vi "Introduce Delay.vi"(8 "error in (no error)":errorcluster, 11 "Ms":u32=100) -> (0 "error out":errorcluster)   [LabVIEW 2018]
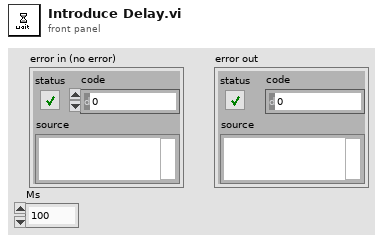
[diagram p1: front panel]
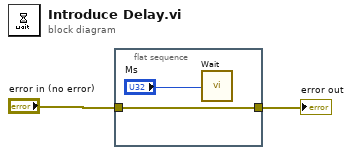
[diagram p0: block diagram]
diagram:
  n1 = flat-sequence {
    tunnel: "error in (no error)" -> [w3]
    tunnel: [w3] -> w2
    frame #0 {
      n2 = call "Wait"("Count(mSec)"="Ms") -> ()  [unwired: 1 out]
    }
  }
  "error out" <- w2
